vi "Re-register for SV Value Update Notification.vi"(8 "error in (no error)":errorcluster, 11 "Father of all uServices in":refnum<class "Father of all uServices.lvclass">) -> (0 "error out":errorcluster, 3 "Father of all uServices out":refnum<class "Father of all uServices.lvclass">)   [LabVIEW 2020, in "TALOS.lvlib" / "Father of all uServices.lvlib" / "Father of all uServices.lvclass"]
doc: "With this VI the uService is asked to re-register for the notifications of the Value Update for the SVs indicated in the corresponding file (more on this later). Useful when the SV to register to get deployed after the uService has started."
uses:
  Father of all uServices.lvclass
  C:/Users/marco/Documents/GitHub_Lab/TALOS/builds/Actor Framework PPL/Actor Framework.lvlibp/1abvi3w/vi.lib/ActorFramework/Actor/Actor.lvclass
  Msg to uServ Selector.ctl
  Father of all uServices Messages/Internal Message to uService Actor Core Msg/Internal Message to uService Actor Core Msg.lvclass/Internal Message to uService Actor Core Msg.ctl
  Ancestor/Ancestor/Ancestor.lvclass/Ancestor.ctl
  Support VIs/Generate Error.vi
  FGV/Error Memory/Get Error Description.vi
  Support VIs/Get PC name.vi
  Ancestor/Ancestor/Read ID.vi
  Support VIs/Get Class Name.vi
  <vilib>/Utility/error.llb/Clear Errors.vi
  FGV/Error Memory/Error Memory Core.vi
  <vilib>/AdvancedString/Delimited String to 1D String Array.vi
  Support VIs/Circus Root Path.vi
  FGV/Error Memory/Error Crt Lvl checker.vi
  FGV/Error Memory/Error Memory Core.vi/40c8088d-b597-4017-91af-faa98e00292e.vi
  FGV/Error Memory/Error Memory Core.vi/d4a3ab98-063c-4e44-b43d-fbdcfe6c2be2.vi
  builds/Actor Framework PPL/Actor Framework.lvlibp/1abvi3w/vi.lib/ActorFramework/Message Enqueuer/Enqueue.vi
  Support VIs/Global Memory.vi
  <vilib>/Utility/LVClass/Get LV Class Name.vi
  Support VIs/Is in Packed Library.vi
  Support VIs/TALOS Root path.vi
  Support VIs/Read CSV worksheet.vi
  Support VIs/Global Constants.vi
  <vilib>/Utility/error.llb/General Error Handler.vi
  Support VIs/Error Log.vi
  Father of all uServices Messages/Internal Message to uService Actor Core Msg/Internal Message to uService Actor Core Msg.lvclass
  Ancestor/Ancestor/Ancestor.lvclass
  <vilib>/Comparison/Equal/Equal Functor/Equal Functor.lvclass
  builds/Actor Framework PPL/Actor Framework.lvlibp/1abvi3w/vi.lib/ActorFramework/Actor/Actor.lvclass
  TALOS.lvlib
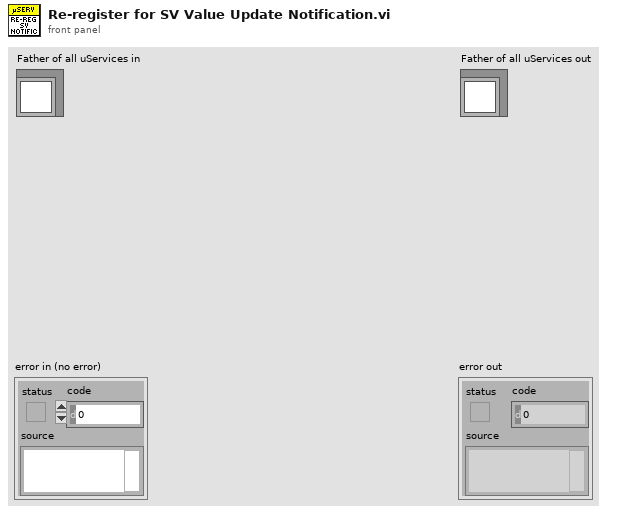
[diagram p1: front panel]
types:
  T1 = typedef "TALOS.lvlib/Father of all uServices.lvlib/Father of all uServices.lvclass/Msg to uServ Selector.ctl" = enum16{"Re-register SV Notification"}
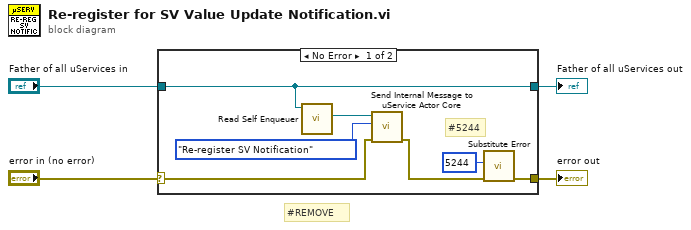
[diagram p0: block diagram]
diagram:
  # "#REMOVE"
  n1 = case shown="No Error" "error in (no error)" {
    selector: "error in (no error)" -> [w10 w13]
    tunnel: [w6 w13] -> w3
    tunnel: [w11 w12] -> w1
    tunnel: "Father of all uServices in" -> [w11 w12]
    frame No Error {
      # "#5244"
      n2 = call "Read Self Enqueuer.vi"("Actor"=w11) -> ("Self Enqueuer"=w8:refnum<class "Message Enqueuer.lvclass">)  [unwired: 10 in]
      n3 = call "Send Internal Message to uService Actor Core.vi"("error in (no error)"=w10, "Msg Selector"=Msg_to_uServ_Selector."Re-register SV Notification", "Message Enqueuer"=w8) -> ("error out"=w5:errorcluster)  [unwired: 7 in, 1 out]
      n4 = call "Substitute Error.vi"("error in (no error)"=w5, "Error Code"=5244) -> ("error out"=w6:errorcluster)  [unwired: 9 in]
    }
    frame Error {
    }
  }
  "error out" <- w3
  "Father of all uServices out" <- w1
